vi "Spectrum_getMapFunction.vi"(0 "MapFunction":T1 items=["Total"=0, "Peak"=4, "Area"=2, "Value"=1, "Ratio"=3]) -> (1 "CursorNames":string[](array[string]), 2 "Function":string)   [LabVIEW 2010]
uses:
  _TypeDefs/MapFunctions.ctl
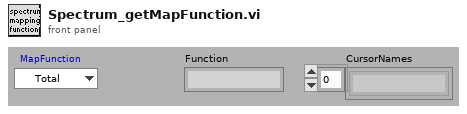
[diagram p1: front panel]
types:
  T1 = typedef "MapFunctions.ctl" = u16
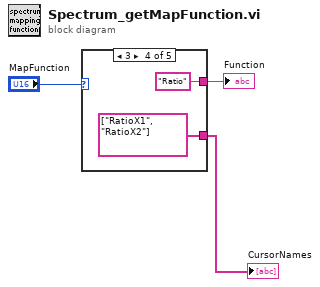
[diagram p0: block diagram]
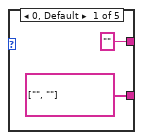
[diagram p2: hidden frame]
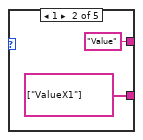
[diagram p3: hidden frame]
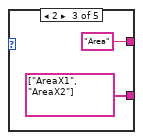
[diagram p4: hidden frame]
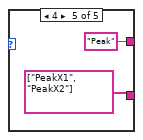
[diagram p5: hidden frame]
diagram:
  n1 = case shown="3" "MapFunction" {
    tunnel: ["" "Value" "Area" "Ratio" "Peak"] -> w1
    tunnel: [string[] ["", ""] string[] ["ValueX1"] string[] ["AreaX1", "AreaX2"] string[] ["RatioX1", "RatioX2"] string[] ["PeakX1", "PeakX2"]] -> w2
    frame 0, Default {
    }
    frame 1 {
    }
    frame 2 {
    }
    frame 3 {
    }
    frame 4 {
    }
  }
  "CursorNames" <- w2
  "Function" <- w1
